vi "Class - By List.vi"(7 "Msg Chain":string, 8 "error in (no error)":errorcluster {"code" format="Error %.0f"}, 10 "Classes":refnum<class "Class Documentation.lvclass">[](array[class]), 11 "VIDoc Printer - Confluence In":refnum<class "VIDoc Printer - Confluence.lvclass">) -> (0 "error out":errorcluster {"code" format="Error %.0f"}, 3 "VIDoc Printer - Confluence Out":refnum<class "VIDoc Printer - Confluence.lvclass">)   [LabVIEW 2023, in "VIDoc Printer - Confluence.lvlib" / "VIDoc Printer - Confluence.lvclass"]
uses:
  VIDoc Printer - Confluence.lvclass
  C:/projects/DMC/Tooling/Git-Action-Service/Source/Documentation Generation/Printers/Printer/VIDoc Printer.lvclass
  Parsing/Class Documentation/Class Documentation.lvclass
  Confluence Formatting/Types/Format Combo Box.ctl
  Printer/VIDoc Printer.lvclass/VIDoc Printer.ctl
  VIDoc Printer - Confluence.lvclass/VIDoc Printer - Confluence.ctl
  Parsing/Class Documentation/Class Documentation.lvclass/Class Documentation.ctl
  Parsing/Class Documentation/Get Class_Library.vi
  Printer/Accessors/Get Class Settings - List Detail Level.vi
  Accessors/Get Class By List Expand.vi
  Confluence Formatting/Confluence Formatting.lvlib
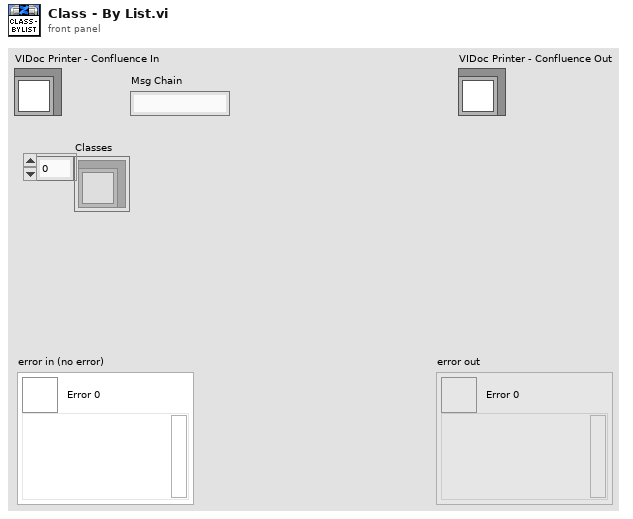
[diagram p1: front panel]
types:
  T1 = typedef "Confluence Formatting.lvlib/Format Combo Box.ctl" = string
  T2 = typedef "VIDoc Printer.lvlib/Printer Settings.lvclass/Detail Level Enum.ctl" = enum16{"None", "Minimal", "Standard", "Full"}
  T3 = typedef "VIDoc Parsing.lvlib/Base Class Info Cluster.ctl" = cluster{"Name":string, "Icon":T4, "Version":cluster{"Major":u16, "Minor":u16, "Fix":u16, "Build":u16}, "Description":string, "Friends":string[], "ChildRefsRestricted":bool, "TransferMustOverrides":bool, "Path":path, "Qualified Name":string, "Class Scope":enum32{"invalid scope", "public", "private", "protected", "community"}}
  T4 = typedef "imagedata.ctl" = cluster{"image type":i32, "image depth":i32, "image":u8[], "mask":u8[], "colors":u32[], "Rectangle":cluster{"left":i16, "top":i16, "right":i16, "bottom":i16}}
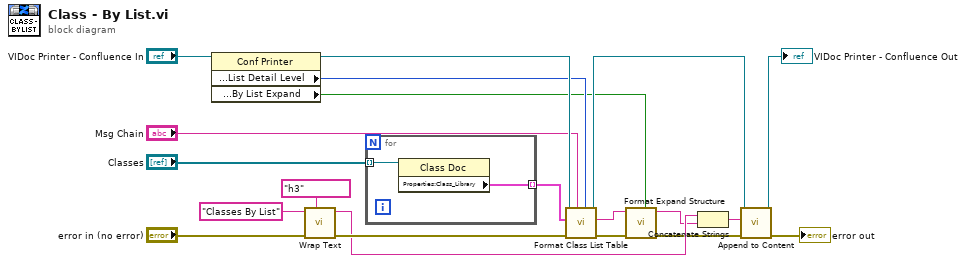
[diagram p0: block diagram]
diagram:
  n1 = property class="Conf Printer"(reference="VIDoc Printer - Confluence In") -> (reference out=w15:refnum<class "VIDoc Printer - Confluence.lvclass">, "Properties:Settings:Classes:List Detail Level"=w2:T2, "Properties:Expand?:Class:By List Expand"=w1:bool)  [unwired: 1 in, 1 out]
  n2 = call "Wrap Text.vi"("Formatting"=T1 "h3", "Error in"="error in (no error)", "String"="Classes By List") -> ("Error out"=w16:errorcluster, "Wrapped String"=w9:string)  [unwired: 7 in]
  n3 = for {
    tunnel: "Classes" -> [w22] mode=indexing
    tunnel: [w21] -> w3 mode=indexing
    n4 = property class="Class Doc"(reference=w22) -> ("Properties:Class_Library"=w21:T3)  [unwired: 1 in, 2 out]
  }
  n5 = call "Format Class List Table.vi"("Detail Level"=w2, "Msg Chain in"="Msg Chain", "error in (no error)"=w16, "Class Info Array"=w3, "VIDoc Printer - Confluence In"=w15) -> ("error out"=w7:errorcluster, "Table Text"=w5:string, "VIDoc Printer - Confluence Out"=w12:refnum<class "VIDoc Printer - Confluence.lvclass">)  [unwired: 4 in]
  n6 = call "Format Expand Structure.vi"("Enable? (T)"=w1, "Error in"=w7, "Content"=w5) -> ("Error out"=w6:errorcluster, "Expand String"=w4:string)  [unwired: 7 in]
  n7 = Concatenate Strings(w9, w4) -> (w14:string)
  n8 = call "Append to Content.vi"("error in (no error)"=w6, "Content"=w14, "VIDoc Printer - Confluence In"=w12) -> ("error out"=→"error out":errorcluster, "VIDoc Printer - Confluence Out"=→"VIDoc Printer - Confluence Out":refnum<class "VIDoc Printer - Confluence.lvclass">)  [unwired: 7 in]
